vi "UART Initialize.vi"(0 "UART Driver in":refnum<class "UART Driver.lvclass">, 5 "RIO Device Name":string, 7 "Number of Ports":u8, 11 "error in":errorcluster) -> (4 "UART Driver out":refnum<class "UART Driver.lvclass">, 15 "error out":errorcluster)   [LabVIEW 2012, in "UART_Host_Driver.lvlib" / "UART Driver.lvclass"]
doc: "Start executing the UART FPGA personality."
uses:
  UART Driver.lvclass
  UART Driver.lvclass/UART Driver.ctl
  <vilib>/FPGAPlugInAG/PXIe-7966R/niLvFpga_Open_PXIe-7966R.vi
  <vilib>/rvi/interface/common/dynamic/niFpgaDynamicAddResources.vi
  <vilib>/rvi/interface/nirviOpenFPGA/nirviOpenFPGA.xnode
  FPGA/builds/UART_Firmware_MultiUp_Debug_0.lvbitx
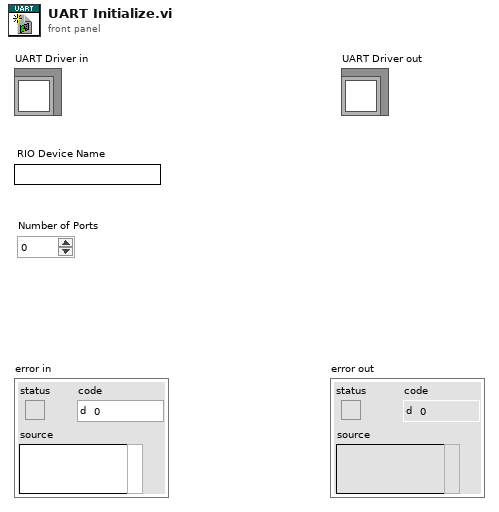
[diagram p1: front panel]
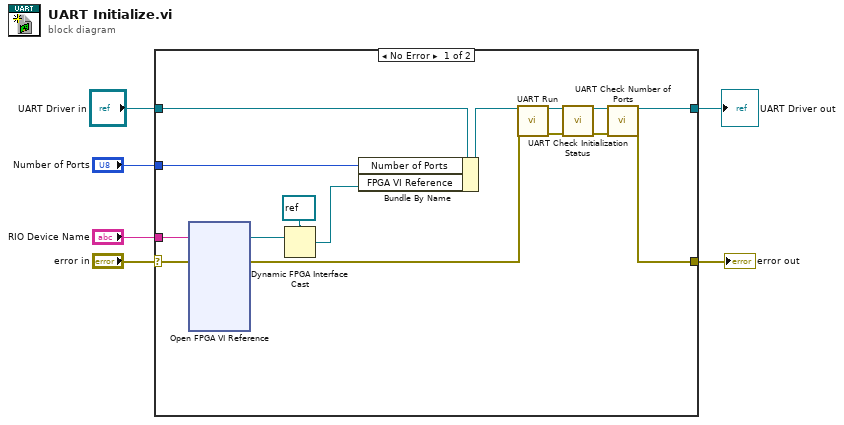
[diagram p0: block diagram]
diagram:
  n1 = case shown="No Error" "error in" {
    selector: "error in" -> [w19 w23]
    tunnel: [w7 w23] -> w5
    tunnel: [w8 w22] -> w3
    tunnel: "UART Driver in" -> [w16 w22]
    tunnel: "RIO Device Name" -> [w18 _]
    tunnel: "Number of Ports" -> [w15 _]
    frame No Error {
      n2 = xnode "Open FPGA VI Reference"("error in"=w19, "resource name"=w18) -> ("FPGA VI Reference Out"=w21:refnum<k20>, "error out"=w13:errorcluster)
      n3 = Dynamic FPGA Interface Cast(Session In=refnum<k20> refnum ("FPGA VI Reference Out"), Type=w21) -> (Session Out=w17:refnum<k20>)
      n4 = Bundle By Name(cluster=w16, "Number of Ports"=w15, "FPGA VI Reference"=w17) -> (w14:refnum<class "UART Driver.lvclass">)
      n5 = call "UART Run.vi"("UART Driver in"=w14, "error in"=w13) -> ("UART Driver out"=w12:refnum<class "UART Driver.lvclass">, "error out"=w11:errorcluster)  [unwired: 12 in]
      n6 = call "UART Check Initialization Status.vi"("UART Driver in"=w12, "error in"=w11) -> ("UART Driver out"=w10:refnum<class "UART Driver.lvclass">, "error out"=w9:errorcluster)  [unwired: 12 in]
      n7 = call "UART Check Number of Ports.vi"("UART Driver in"=w10, "error in"=w9) -> ("UART Driver out"=w8:refnum<class "UART Driver.lvclass">, "error out"=w7:errorcluster)  [unwired: 12 in]
    }
    frame Error {
    }
  }
  "error out" <- w5
  "UART Driver out" <- w3
